vi "get_predefined_commands.vi"(8 "error in (no error)":errorcluster, 10 "value_to_set":u32, 11 "Predefined_routines":T2="decommissioning") -> (0 "error out":errorcluster, 1 "addressings":T1[](array[typedef]), 2 "data":u32[](array[numeric]) format="%x", 3 "commands":u32[](array[numeric]))   [LabVIEW 2014, in "Driver_interaction.lvlib" / "Dali_usb_tridonics.lvclass"]
uses:
  Dali_usb_tridonics.lvclass
  Controls/Predefined_routines.ctl
  Vendor/Controls/Addressing_type.ctl
  Deploy/Utilities/Miscelanous.lvlibp/Controls/Configuration_file.ctl
  <vilib>/Utility/file.llb/Read From Spreadsheet File (string).vi
  Deploy/Utilities/Miscelanous.lvlibp
  Vendor/Dali_usb.lvlib
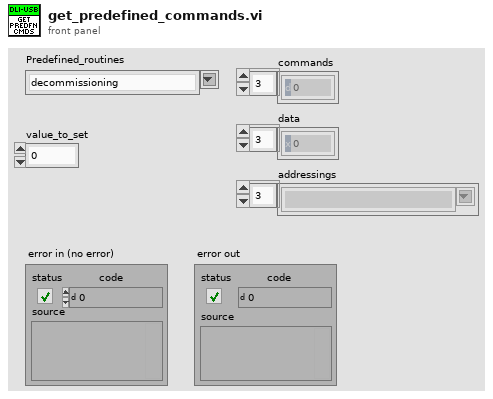
[diagram p1: front panel]
types:
  T1 = typedef "Dali_usb.lvlib/Addressing_type.ctl" = string
  T2 = typedef "Driver_interaction.lvlib/Dali_usb_tridonics.lvclass/Predefined_routines.ctl" = string
  T3 = typedef "Miscelanous.lvlibp/Configuration_file.ctl" = enum16{"Station_settings", "Instrument_config", "Test_config", "Error_log", "Vision_maintenance", "Services", "Mapping_signals", "Failures", "JOT_firmware", "Station_settings_template", "PLC_signals_by_firmware"}
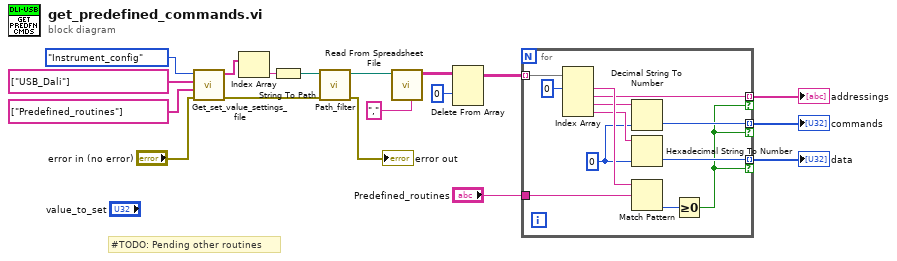
[diagram p0: block diagram]
diagram:
  # "#TODO: Pending other routines"
  n1 = call "Get_set_value_settings_file.vi"("error in"="error in (no error)", "keys"=string[] ["Predefined_routines"] ("sections"), "sections"=string[] ["USB_Dali"], "Configuration file"=Configuration_file."Instrument_config") -> ("error out"=w3:errorcluster, "values out"=w7:string[])  [unwired: 6 in]
  n2 = Index Array(array=w7) -> (element=w6:string)  [unwired: 1 in]
  n3 = String To Path(string=w6) -> (path=w5:path)
  n4 = call "Path_filter.vi"("error in (no error)"=w3, "Path_unfiltered"=w5) -> ("error out"=→"error out":errorcluster, "Path_filtered"=w4:path)  [unwired: 8 in]
  n5 = call-poly <vilib>:"Read From Spreadsheet File.vi"("delimiter (\\t)"="," ("delimiter (\\t)"), "file path (dialog if empty)"=w4) -> ("all rows"=w17:string[][])  [unwired: 5 in, 4 out]
  n6 = Delete From Array(array=w17, index (row)=0 ("disabled index (col)")) -> (array with subset deleted=w15:string[][])  [unwired: 2 in, 1 out]
  n7 = for {
    tunnel: w15 -> [w30] mode=indexing
    tunnel: "Predefined_routines" -> [w27]
    tunnel: [w25] -> w12 mode=indexing if=w20
    tunnel: [w24] -> w13 mode=indexing if=w20
    tunnel: [w21] -> w11 mode=indexing if=w20
    w19 = u32 0 ("default (0 I32)")
    n8 = Index Array(array=w30, index #1=0 ("index")) -> (element #1=w28:string, element #2=w24:string, element #3=w26:string, element #4=w22:string)  [unwired: 3 in]
    n9 = Decimal String To Number(string=w26, default (0L)=w19) -> (number=w25:u32)  [unwired: 1 in, 1 out]
    n10 = Hexadecimal String To Number(string=w22, default (0uL)=w19) -> (number=w21:u32)  [unwired: 1 in, 1 out]
    n11 = Match Pattern(string=w28, regular expression=w27) -> (offset past match=w23:i32)  [unwired: 1 in, 3 out]
    n12 = Greater Or Equal To 0?(x=w23) -> (x >= 0?=w20:bool)
  }
  "commands" <- w12
  "addressings" <- w13
  "data" <- w11
